vi "JoyScale.vi"(1 "Max Power":dbl, 2 "DeadZone":dbl, 3 "JoyValue":dbl) -> (0 "Motor Value":dbl)   [LabVIEW 2011]
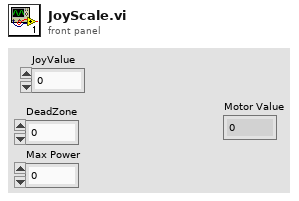
[diagram p1: front panel]
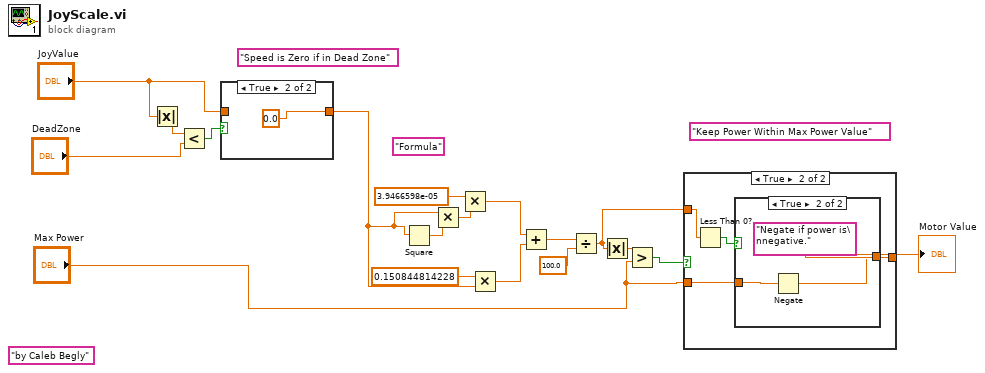
[diagram p0: block diagram]
diagram:
  (unwired) "by Caleb Begly"
  (unwired) "Keep Power Within Max Power Value"
  (unwired) "Speed is Zero if in Dead Zone"
  (unwired) "Formula"
  n1 = Absolute Value(x="JoyValue") -> (abs(x)=w10:dbl)
  n2 = Less?(x=w10, y="DeadZone") -> (x < y?=w9:bool)
  n3 = case shown="True" w9 {
    tunnel: "JoyValue" -> [w19 _]
    tunnel: [w19 0.0 ("JoyValue")] -> w6
    frame False {
    }
    frame True {
    }
  }
  n4 = Square(x=w6) -> (x^2=w18:dbl)
  n5 = Multiply(x=w6, y=w18) -> (x*y=w17:dbl)
  n6 = Multiply(x=3.9466598e-05, y=w17) -> (x*y=w15:dbl)
  n7 = Multiply(x=0.150844814228, y=w6) -> (x*y=w14:dbl)
  n8 = Add(x=w15, y=w14) -> (x+y=w12:dbl)
  n9 = Divide(x=w12, y=100.0) -> (x/y=w1:dbl)
  n10 = Absolute Value(x=w1) -> (abs(x)=w2:dbl)
  n11 = Greater?(x=w2, y="Max Power") -> (0:w5:bool)
  n12 = case shown="True" w5 {
    tunnel: "Max Power" -> [_ w23]
    tunnel: [w21 w22] -> w3
    tunnel: w1 -> [w21 w25]
    frame False {
    }
    frame True {
      n13 = Less Than 0?(x=w25) -> (x < 0?=w24:bool)
      n14 = case shown="True" w24 {
        tunnel: w23 -> [w26 w28]
        tunnel: [w26 w27] -> w22
        frame False {
        }
        frame True {
          (unwired) "Negate if power is\nnegative."
          n15 = Negate(x=w28) -> (-x=w27:dbl)
        }
      }
    }
  }
  "Motor Value" <- w3
